vi "Calculate Linearity.vi"(8 "error in (no error)":errorcluster, 9 "SensorID":i32, 10 "FS Sensors":T2[](array[typedef]), 11 "Sorted Calibration Points":T3[][](array[typedef])) -> (0 "error out":errorcluster, 3 "Linearity Results":T1[](array[typedef]))   [LabVIEW 2026, in "Analysis.lvlib"]
uses:
  Analysis.lvlib
  controls/Messaging Payloads/Calibration Point Table Insert.ctl
  Full Scale Sensor Cluster.ctl
  Linearity Result.ctl
  <vilib>/Analysis/NI_AALPro.lvlib
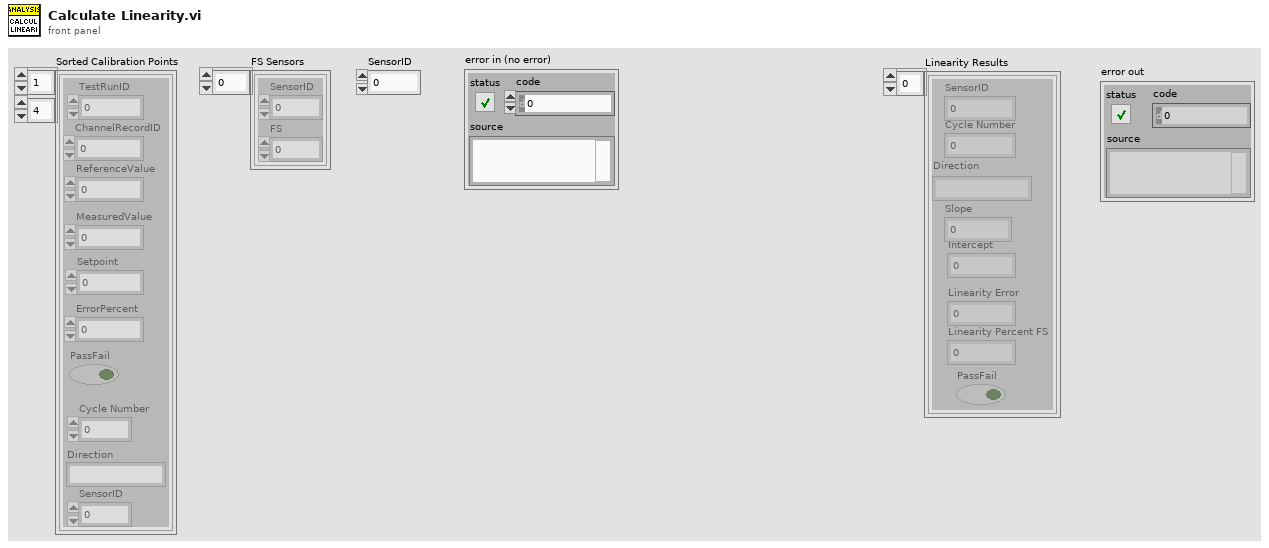
[diagram p1: front panel]
types:
  T1 = typedef "Analysis.lvlib/Linearity Result.ctl" = cluster{"Slope":dbl, "Intercept":dbl, "Cycle Number":i32, "SensorID":i32, "Linearity Error":dbl, "Linearity Percent FS":dbl, "Direction":string, "PassFail":bool}
  T2 = typedef "Analysis.lvlib/Full Scale Sensor Cluster.ctl" = cluster{"SensorID":i32, "FS":dbl}
  T3 = typedef "Calibration Point Table Insert.ctl" = cluster{"TestRunID":i32, "ChannelRecordID":i32, "Setpoint":dbl, "MeasuredValue":dbl, "ErrorPercent":dbl, "PassFail":bool, "ReferenceValue":dbl, "Cycle Number":i32, "Direction":string, "SensorID":i32}
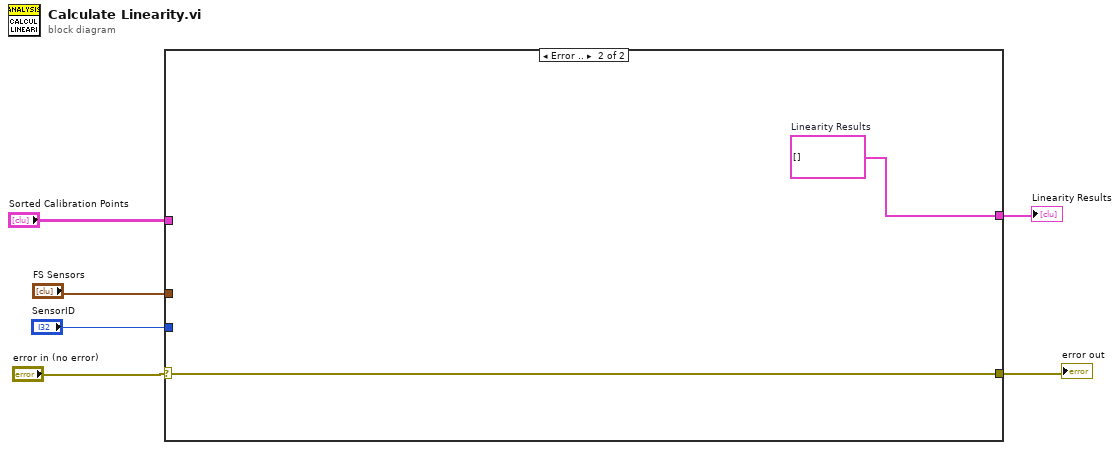
[diagram p0: block diagram]
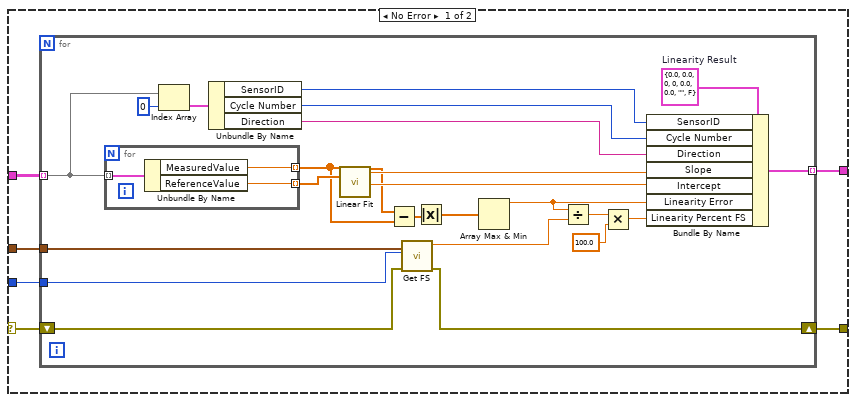
[diagram p2: hidden frame]
diagram:
  n1 = case shown="Error .." "error in (no error)" {
    selector: "error in (no error)" -> [w11 w41]
    tunnel: "Sorted Calibration Points" -> [w12 _]
    tunnel: [w10 w41] -> w4
    tunnel: "FS Sensors" -> [w9 _]
    tunnel: [w8 w40] -> w2
    tunnel: "SensorID" -> [w7 _]
    frame No Error {
      n2 = for {
        tunnel: w12 -> [w23] mode=indexing
        tunnel: [w36] -> w8 mode=indexing
        tunnel: w9 -> [w18]
        shift-right: [w14] -> w10
        shift-left: w11 -> [w15]
        tunnel: w7 -> [w13]
        w35 = T1 {"Slope"=0.0, "Intercept"=0.0, "Cycle Number"=0, "SensorID"=0, "Linearity Error"=0.0, "Linearity Percent FS"=0.0, "Direction"="", "PassFail"=FALSE}  # Linearity Result
        n3 = for {
          tunnel: w23 -> [w37] mode=indexing
          tunnel: [w39] -> w31 mode=indexing
          tunnel: [w38] -> w34 mode=indexing
          n4 = Unbundle By Name(w37) -> ("MeasuredValue"=w39:dbl, "ReferenceValue"=w38:dbl)
        }
        n5 = Index Array(array=w23, index=0) -> (element=w22:T3)
        n6 = Unbundle By Name(w22) -> ("SensorID"=w16:i32, "Cycle Number"=w20:i32, "Direction"=w19:string)
        n7 = call <vilib>:"Linear Fit.vi"("Y"=w31, "X"=w34) -> ("Best Linear Fit"=w30:dbl[], "slope"=w33:dbl, "intercept"=w32:dbl)  [unwired: 9 in, 2 out]
        n8 = Subtract(x=w30, y=w31) -> (x-y=w29:dbl[])
        n9 = call "Get FS.vi"("error in (no error)"=w15, "SensorID"=w13, "FS Sensors"=w18) -> ("error out"=w14:errorcluster, "FS"=w17:dbl)  [unwired: 7 in]
        n10 = Absolute Value(x=w29) -> (abs(x)=w26:dbl[])
        n11 = Array Max & Min(array=w26) -> (max value=w25:dbl)  [unwired: 3 out]
        n12 = Divide(x=w25, y=w17) -> (x/y=w28:dbl)
        n13 = Multiply(x=w28, y=100.0) -> (x*y=w21:dbl)
        n14 = Bundle By Name(cluster=w35, "SensorID"=w16, "Cycle Number"=w20, "Direction"=w19, "Slope"=w33, "Intercept"=w32, "Linearity Error"=w25, "Linearity Percent FS"=w21) -> (w36:T1)
      }
    }
    frame Error {
      w40 = T1[] []  # Linearity Results
    }
  }
  "error out" <- w4
  "Linearity Results" <- w2
